vi "Multi_Stop_Button.vi"() -> ()   [LabVIEW 2023]
panel:
  in  "Stop Button":bool
  out "Waveform Graph 2":dbl[][](graph)
  out "Waveform Graph":dbl[][](graph)
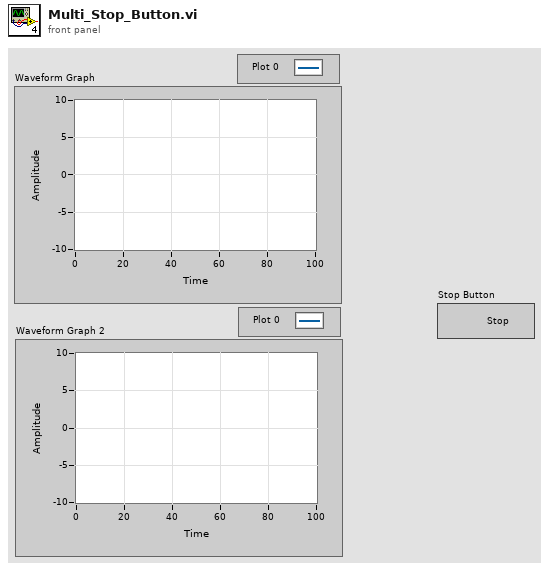
[diagram p1: front panel]
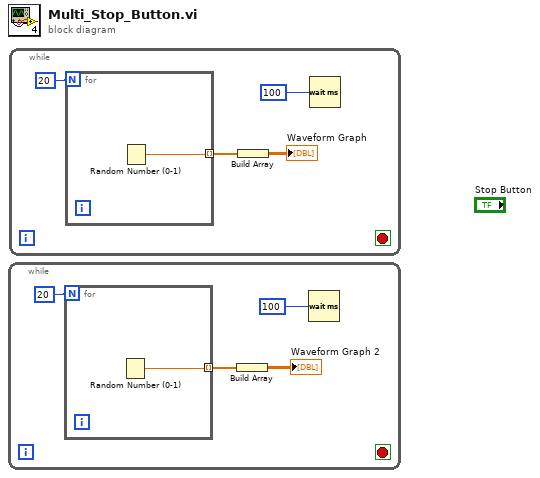
[diagram p0: block diagram]
diagram:
  n1 = while {
    stop <- _ stop-if-true
    n2 = for {
      N: 20 -> [_]
      tunnel: [w5] -> w3 mode=indexing
      n3 = Random Number (0-1)() -> (number: 0 to 1=w5:dbl)
    }
    n4 = Build Array(w3) -> (→"Waveform Graph 2":dbl[][])
    n5 = Wait (ms)(milliseconds to wait=u32 100) -> ()  [unwired: 1 out]
  }
  n6 = while {
    stop <- _ stop-if-true
    n7 = for {
      N: 20 -> [_]
      tunnel: [w10] -> w8 mode=indexing
      n8 = Random Number (0-1)() -> (number: 0 to 1=w10:dbl)
    }
    n9 = Build Array(w8) -> (→"Waveform Graph":dbl[][])
    n10 = Wait (ms)(milliseconds to wait=u32 100) -> ()  [unwired: 1 out]
  }
